vi "MusicLoop.vi"(8 "error in (no error)":errorcluster, 10 "Tracks":path, 11 "Engine in":refnum<class "Engine.lvclass">) -> (0 "error out":errorcluster)   [LabVIEW 2019, in "RT_Game.lvlib" / "Engine.lvclass"]
uses:
  Engine.lvclass
  MusicLoopData.ctl
  Engine.lvclass/Engine.ctl
  Game/Game.lvclass/Game.ctl
  ChangeVolumeData.ctl
  Game/Read FPGA_ref.vi
  <vilib>/Utility/error.llb/Error Cluster From Error Code.vi
  <vilib>/rvi/errors/niLvFpgaAdjustHostInterfaceError.vi
  <vilib>/rvi/interface/common/niFpgaWaitOnOcc.vi
  FPGA_Interface.ctl
  <vilib>/rvi/interface/nirviMethod/nirviMethod.xnode
  FPGA Bitfiles/myriogameconsole_FPGATarget_Main_ntsPRcBZGxk.lvbitx
  <vilib>/FPGAPlugInAG/myRIO-1900/niLvFpga_WriteFifo_myRIO-1900.vi
  <vilib>/rvi/errors/niLvFpgaMergeErrorWithErrorCode.vi
  <vilib>/FPGAPlugInAG/myRIO-1900/niLvFpga_ConfigureFifo_myRIO-1900.vi
  Game/Game.lvclass
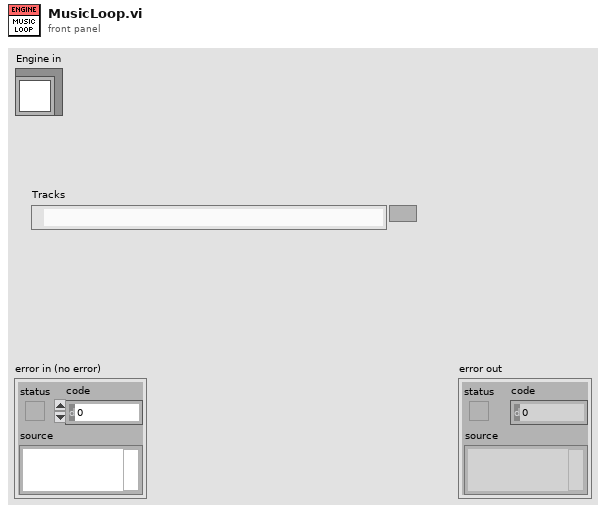
[diagram p1: front panel]
types:
  T1 = typedef "RT_Game.lvlib/Engine.lvclass/MusicLoopData.ctl" = cluster{"Music":i16[], "Position":u32, "ActualDepth":u32, "PackageSize":i32, "FileRefnum":refnum<file>, "Volume":dbl, "WaitTime":i32}
  T2 = typedef "RT_Game.lvlib/Engine.lvclass/ChangeVolumeData.ctl" = enum16{"up", "down", "mute"}
  T3 = typedef "FPGA_Interface.ctl" = refnum<k20>
  T4 = typedef "RT_Game.lvlib/Engine.lvclass/MessageCluster.ctl" = cluster{"Message":string, "Data":variant}
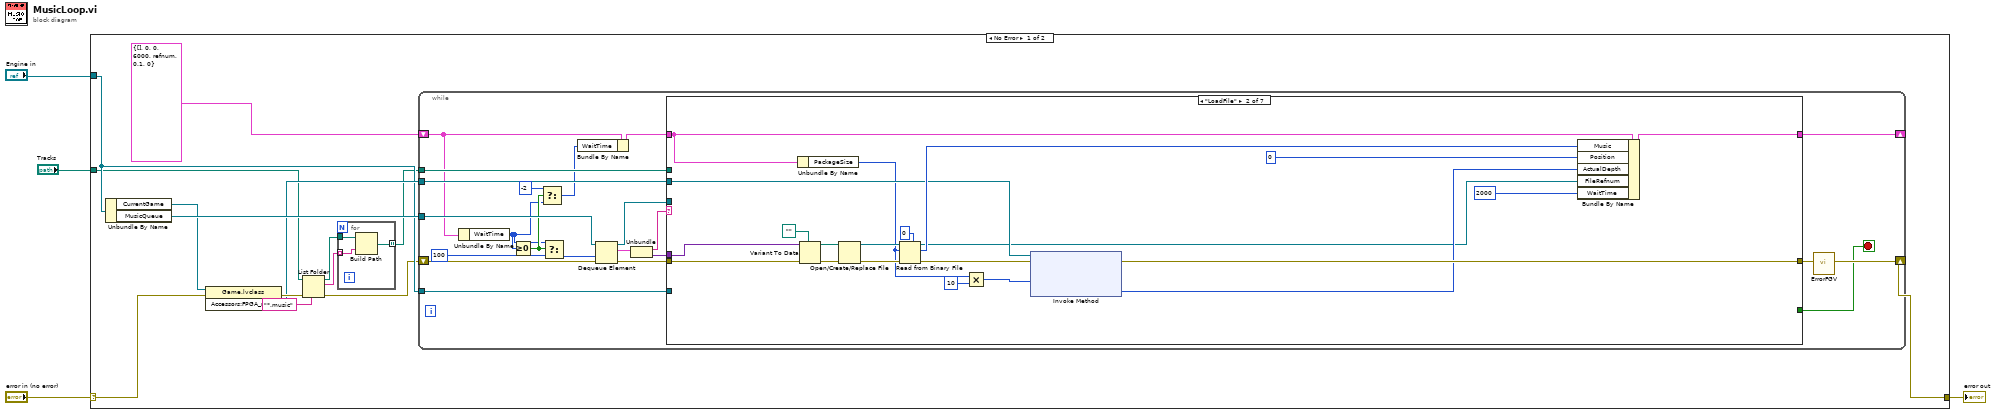
[diagram p0: block diagram]
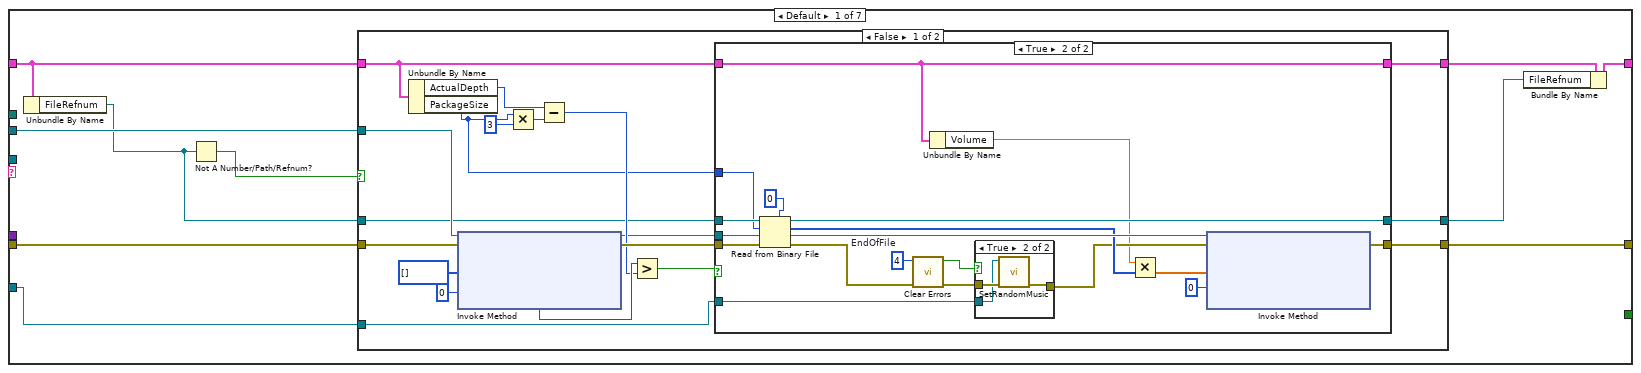
[diagram p2: hidden frame]
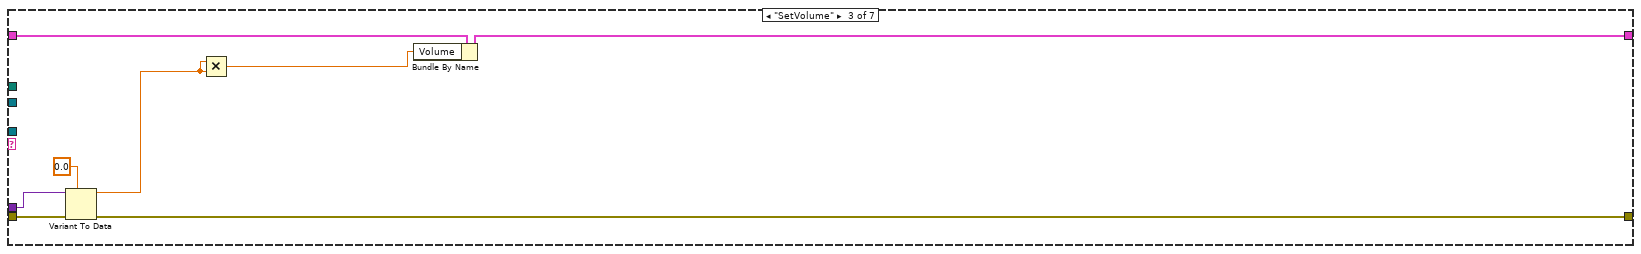
[diagram p6: hidden frame]
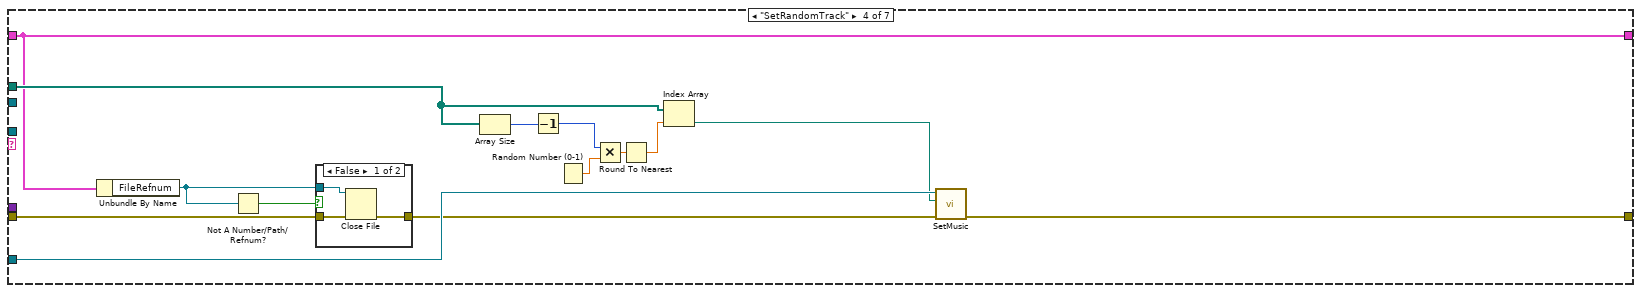
[diagram p7: hidden frame]
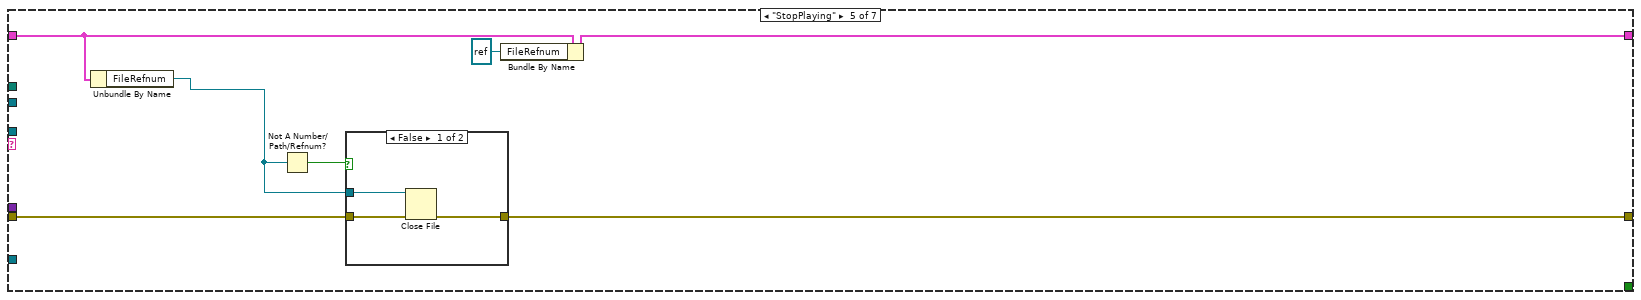
[diagram p9: hidden frame]
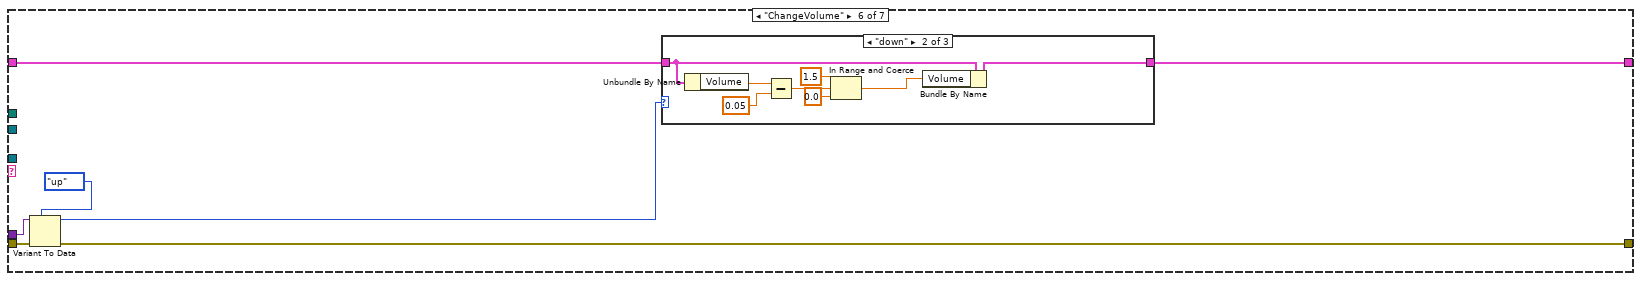
[diagram p11: hidden frame]
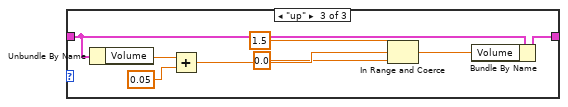
[diagram p13: hidden frame]
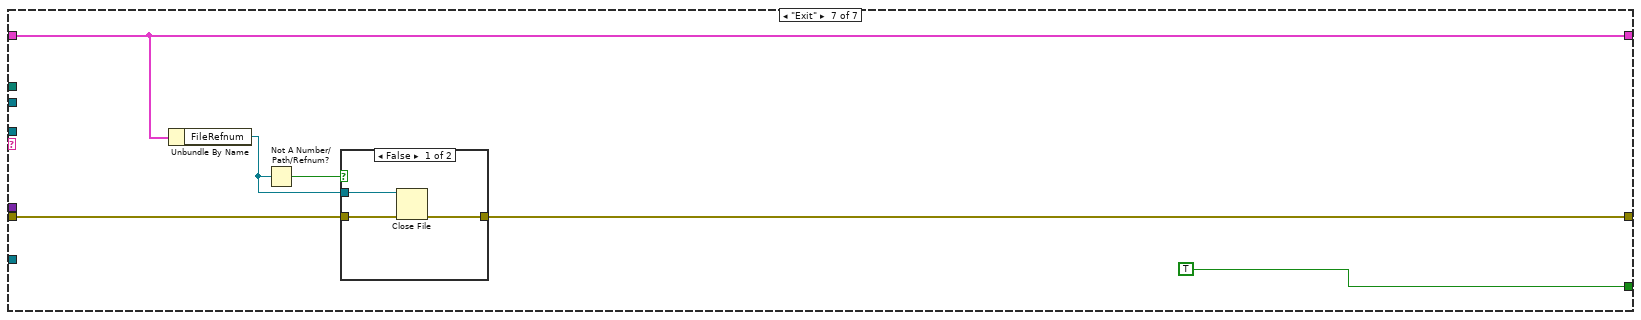
[diagram p14: hidden frame]
diagram:
  n1 = case shown="No Error" "error in (no error)" {
    selector: "error in (no error)" -> [w18 w193]
    tunnel: [w17 w193] -> w3
    tunnel: "Engine in" -> [w11 _]
    tunnel: "Tracks" -> [w8 _]
    frame No Error {
      n2 = Unbundle By Name(w11) -> ("CurrentGame"=w13:refnum<class "Game.lvclass">, "MusicQueue"=w16:refnum<queue>)
      n3 = property class="Game.lvclass"(reference=w13, error in=w18) -> (error out=w14:errorcluster, "Accessors:FPGA_ref"=w12:T3)  [unwired: 1 out]
      n4 = List Folder(path=w8, pattern="*.music", error in=w14) -> (path out=w7:path, filenames=w6:string[], error out=w10:errorcluster)  [unwired: 1 in, 1 out]
      n5 = for {
        tunnel: w7 -> [w21]
        tunnel: w6 -> [w20] mode=indexing
        tunnel: [w19] -> w5 mode=indexing
        n6 = Build Path(base path=w21, name or relative path=w20) -> (appended path=w19:path)
      }
      n7 = while {
        shift-right: [w23] -> w17
        shift-left: w10 -> [w43]
        tunnel: w16 -> [w41]
        shift-right: [w37] -> _
        shift-left: T1 {"Music"=[], "Position"=0, "ActualDepth"=0, "PackageSize"=6000, "FileRefnum"=refnum, "Volume"=0.1, "WaitTime"=0} -> [w29]
        tunnel: w12 -> [w35]
        tunnel: w5 -> [w32]
        tunnel: w11 -> [w31]
        stop <- w22 stop-if-true
        n8 = Unbundle By Name(w29) -> ("WaitTime"=w26:i32)
        n9 = Greater Or Equal To 0?(x=w26) -> (x >= 0?=w27:bool)
        n10 = Select(t=-2, s=w27, f=w26) -> (s? t:f=w24:i32)
        n11 = Select(t=w26, s=w27, f=100 ("timeout in ms (-1)")) -> (s? t:f=w30:i32)
        n12 = Bundle By Name(cluster=w29, "WaitTime"=w24) -> (w28:T1)
        n13 = Dequeue Element(queue=w41, timeout in ms (-1)=w30, error in (no error)=w43) -> (queue out=w36:refnum<queue>, element=w40:T4, error out=w42:errorcluster)  [unwired: 1 out]
        n14 = Unbundle(w40) -> ("Message"=w39:string, "Data"=w38:variant)
        n15 = case shown="\"LoadFile\"" w39 {
          tunnel: w42 -> [w53 w121 w129 w143 w154 w165 w188]
          tunnel: [w52 w110 w127 w138 w152 w163 w185] -> w33
          tunnel: w38 -> [_ w119 w126 _ _ w162 _]
          tunnel: [w47 w113 w124 w135 w151 w160 w186] -> w37
          tunnel: w28 -> [w49 w106 w128 w135 w153 w164 w186]
          tunnel: w36 -> [_ _ _ _ _ _ _]
          tunnel: w35 -> [w51 w109 _ _ _ _ _]
          tunnel: [_ _ _ _ _ _ TRUE] -> w22
          tunnel: w32 -> [_ _ _ w140 _ _ _]
          tunnel: w31 -> [w44 _ _ w137 _ _ _]
          frame Default {
            n16 = Unbundle By Name(w49) -> ("FileRefnum"=w48:refnum<file>)
            n17 = Not A Number/Path/Refnum?(number/path/refnum=w48) -> (NaN/Path/Refnum?=w50:bool)
            n18 = case shown="False" w50 {
              tunnel: w53 -> [w72 w99]
              tunnel: [w63 w99] -> w52
              tunnel: w51 -> [w70 _]
              tunnel: w49 -> [w56 w98]
              tunnel: w48 -> [w60 w100]
              tunnel: [w59 w100] -> w46
              tunnel: [w55 w98] -> w45
              tunnel: w44 -> [w54 _]
              frame False {
                n19 = Unbundle By Name(w56) -> ("ActualDepth"=w68:u32, "PackageSize"=w58:i32)
                n20 = xnode "Invoke Method"("FPGA VI Reference In"=w70, "error in"=w72, "Data"=i16[] [], "Timeout (ms)"=0) -> ("FPGA VI Reference Out"=w62:T3, "error out"=w71:errorcluster, "Empty Elements Remaining"=w65:u32)
                n21 = Multiply(x=w58, y=3) -> (x*y=w67:i32)
                n22 = Subtract(x=w68, y=w67) -> (x-y=w64:u32)
                n23 = Greater?(x=w65, y=w64) -> (0:w61:bool)
                n24 = case shown="True" w61 {
                  tunnel: w71 -> [w75 w93]
                  tunnel: [w75 w92] -> w63
                  tunnel: w62 -> [_ w91]
                  tunnel: w60 -> [w74 w89]
                  tunnel: [w74 w79] -> w59
                  tunnel: w58 -> [_ w87]
                  tunnel: [w73 w77] -> w55
                  tunnel: w56 -> [w73 w77]
                  tunnel: w54 -> [_ w78]
                  frame False {
                  }
                  frame True {
                    w83 = 4  # EndOfFile
                    n25 = Read from Binary File(5:i16 0 ("y"), 8:w93, 10:w87, 11:w89) -> (0:w90:errorcluster, 2:w86:i16[], 3:w79:refnum<file>)  [unwired: 2 in, 1 out]
                    n26 = call <vilib>:"Clear Errors.vi"("error in (no error)"=w90, "specific error code to clear (0: all)"=w83) -> ("error out"=w84:errorcluster, "specific error cleared?"=w81:bool)  [unwired: 4 in]
                    n27 = Unbundle By Name(w77) -> ("Volume"=w76:dbl)
                    n28 = case shown="True" w81 {
                      tunnel: w84 -> [w94 w97]
                      tunnel: [w94 w96] -> w82
                      tunnel: w78 -> [_ w95]
                      frame False {
                      }
                      frame True {
                        n29 = call "SetRandomMusic.vi"("error in (no error)"=w97, "Engine in"=w95) -> ("error out"=w96:errorcluster)  [unwired: 8 in, 1 out]
                      }
                    }
                    n30 = Multiply(x=w76, y=w86) -> (x*y=w80:dbl[])
                    n31 = xnode "Invoke Method"("FPGA VI Reference In"=w91, "error in"=w82, "Data"=w80, "Timeout (ms)"=0) -> ("error out"=w92:errorcluster)  [unwired: 2 out]
                  }
                }
              }
              frame True {
              }
            }
            n32 = Bundle By Name(cluster=w45, "FileRefnum"=w46) -> (w47:T1)
          }
          frame "LoadFile" {
            n33 = Unbundle By Name(w106) -> ("PackageSize"=w103:i32)
            n34 = Variant To Data(error in=w121, type=path "", Variant=w119) -> (data=w116:path, error out=w120:errorcluster)
            n35 = Open/Create/Replace File(file path (use dialog)=w116, error in=w120) -> (refnum out=w114:refnum<file>, error out=w117:errorcluster)  [unwired: 4 in, 1 out]
            n36 = Read from Binary File(5:i16 0 ("Music"), 8:w117, 10:w103, 11:w114) -> (0:w115:errorcluster, 2:w112:i16[], 3:w105:refnum<file>)  [unwired: 2 in, 1 out]
            n37 = Multiply(x=w103, y=10) -> (x*y=w101:i32)
            n38 = xnode "Invoke Method"("FPGA VI Reference In"=w109, "error in"=w115, "Requested Depth"=w101) -> ("error out"=w110:errorcluster, "Actual Depth"=w108:u32)  [unwired: 1 out]
            n39 = Bundle By Name(cluster=w106, "Music"=w112, "Position"=u32 0, "ActualDepth"=w108, "FileRefnum"=w105, "WaitTime"=2000) -> (w113:T1)
          }
          frame "SetVolume" {
            n40 = Variant To Data(error in=w129, type=0.0, Variant=w126) -> (data=w122:dbl, error out=w127:errorcluster)
            n41 = Multiply(x=w122, y=w122) -> (x*y=w123:dbl)
            n42 = Bundle By Name(cluster=w128, "Volume"=w123) -> (w124:T1)
          }
          frame "SetRandomTrack" {
            n43 = Unbundle By Name(w135) -> ("FileRefnum"=w132:refnum<file>)
            n44 = Not A Number/Path/Refnum?(number/path/refnum=w132) -> (NaN/Path/Refnum?=w133:bool)
            n45 = case shown="False" w133 {
              tunnel: w143 -> [w146 w147]
              tunnel: [w145 w147] -> w134
              tunnel: w132 -> [w144 _]
              frame False {
                n46 = Close File(refnum=w144, error in=w146) -> (error out=w145:errorcluster)  [unwired: 1 out]
              }
              frame True {
              }
            }
            n47 = Array Size(array=w140) -> (size(s)=w142:i32)
            n48 = Decrement(x=w142) -> (x-1=w131:i32)
            n49 = Random Number (0-1)() -> (number: 0 to 1=w141:dbl)
            n50 = Multiply(x=w131, y=w141) -> (x*y=w139:dbl)
            n51 = Round To Nearest(number=w139) -> (nearest integer value=w130:dbl)
            n52 = Index Array(array=w140, index=w130) -> (element=w136:path)
            n53 = call "SetMusic.vi"("error in (no error)"=w134, "Path"=w136, "Engine in"=w137) -> ("error out"=w138:errorcluster)  [unwired: 7 in, 1 out]
          }
          frame "StopPlaying" {
            n54 = Unbundle By Name(w153) -> ("FileRefnum"=w149:refnum<file>)
            n55 = Not A Number/Path/Refnum?(number/path/refnum=w149) -> (NaN/Path/Refnum?=w148:bool)
            n56 = case shown="False" w148 {
              tunnel: w154 -> [w157 w158]
              tunnel: [w156 w158] -> w152
              tunnel: w149 -> [w155 _]
              frame False {
                n57 = Close File(refnum=w155, error in=w157) -> (error out=w156:errorcluster)  [unwired: 1 out]
              }
              frame True {
              }
            }
            n58 = Bundle By Name(cluster=w153, "FileRefnum"=refnum<file> refnum) -> (w151:T1)
          }
          frame "ChangeVolume" {
            n59 = Variant To Data(error in=w165, type=ChangeVolumeData."up" ("VolumeData"), Variant=w162) -> (data=w159:T2, error out=w163:errorcluster)
            n60 = case shown="\"down\"" w159 {
              tunnel: w164 -> [w166 w173 w181]
              tunnel: [w166 w174 w182] -> w160
              frame "mute", Default {
              }
              frame "down" {
                n61 = Unbundle By Name(w173) -> ("Volume"=w171:dbl)
                n62 = Subtract(x=w171, y=0.05) -> (x-y=w172:dbl)
                n63 = In Range and Coerce(upper limit=1.5, x=w172, lower limit=0.0) -> (coerced(x)=w169:dbl)  [unwired: 1 out]
                n64 = Bundle By Name(cluster=w173, "Volume"=w169) -> (w174:T1)
              }
              frame "up" {
                n65 = Unbundle By Name(w181) -> ("Volume"=w179:dbl)
                n66 = Add(x=w179, y=0.05) -> (x+y=w180:dbl)
                n67 = In Range and Coerce(upper limit=1.5, x=w180, lower limit=0.0) -> (coerced(x)=w177:dbl)  [unwired: 1 out]
                n68 = Bundle By Name(cluster=w181, "Volume"=w177) -> (w182:T1)
              }
            }
          }
          frame "Exit" {
            n69 = Unbundle By Name(w186) -> ("FileRefnum"=w184:refnum<file>)
            n70 = Not A Number/Path/Refnum?(number/path/refnum=w184) -> (NaN/Path/Refnum?=w183:bool)
            n71 = case shown="False" w183 {
              tunnel: w188 -> [w191 w192]
              tunnel: [w190 w192] -> w185
              tunnel: w184 -> [w189 _]
              frame False {
                n72 = Close File(refnum=w189, error in=w191) -> (error out=w190:errorcluster)  [unwired: 1 out]
              }
              frame True {
              }
            }
          }
        }
        n73 = call "ErrorFGV.vi"("error in (no error)"=w33) -> ("error out"=w23:errorcluster)  [unwired: 9 in, 1 out]
      }
    }
    frame Error {
    }
  }
  "error out" <- w3
